vi "Execute.vi"(8 "error in":errorcluster, 10 "Update Settings in":refnum<class "Update Settings.lvclass">, 11 "Object In":refnum<class>) -> (0 "error out":errorcluster, 3 "Object Out":refnum<class>)   [LabVIEW 2014, in "Update Settings.lvclass"]
doc: "Abstract method for accomplishing the execution of a command directed to an instrument object on the wire."
uses:
  Update Settings.lvclass
  Instr Actor.lvclass
  Update Settings.lvclass/Update Settings.ctl
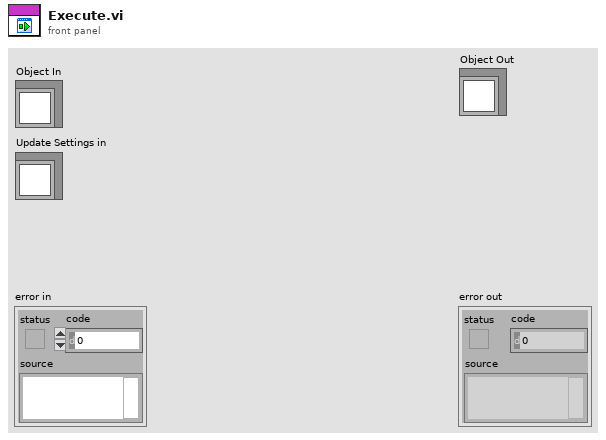
[diagram p1: front panel]
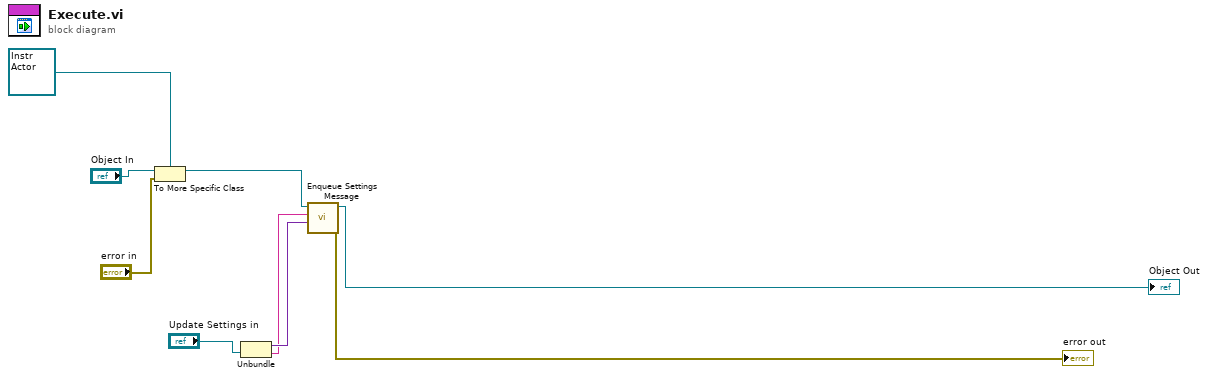
[diagram p0: block diagram]
diagram:
  n1 = To More Specific Class(target class=refnum<class "Instr Actor.lvclass"> refnum ("Instrument Lib:Instr"), reference="Object In", error in="error in") -> (specific class reference=w6:refnum<class "Instr Actor.lvclass">)  [unwired: 1 out]
  n2 = Unbundle("Update Settings in") -> (w4:variant, w3:string)
  n3 = call "Enqueue Settings Message.vi"("Data"=w4, "Key"=w3, "Instr in"=w6) -> ("error out"=→"error out":errorcluster, "Instr out"=→"Object Out":refnum<class "Instr Actor.lvclass">)  [unwired: 7 in]
